vi "Close Log File.vi"(8 "error in (no error)":errorcluster, 11 "PCAP Frame Logger in":refnum<class "PCAP Frame Logger.lvclass">) -> (0 "error out":errorcluster, 3 "PCAP Frame Logger out":refnum<class "PCAP Frame Logger.lvclass">)   [LabVIEW 2020, in "Frame Logging.lvlib" / "PCAP Frame Logger.lvclass"]
uses:
  PCAP Frame Logger.lvclass
  PCAP Frame Logger.lvclass/PCAP Frame Logger.ctl
  <vilib>/Utility/SystemLogging/NI_SystemLogging.lvlib
  libpcaplv/libpcaplv.lvlib
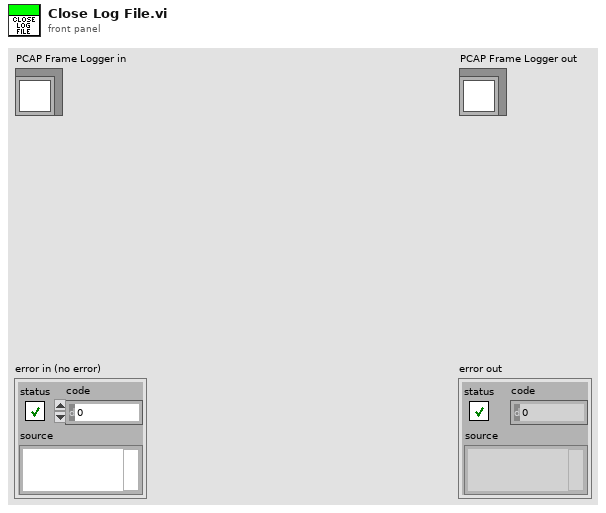
[diagram p1: front panel]
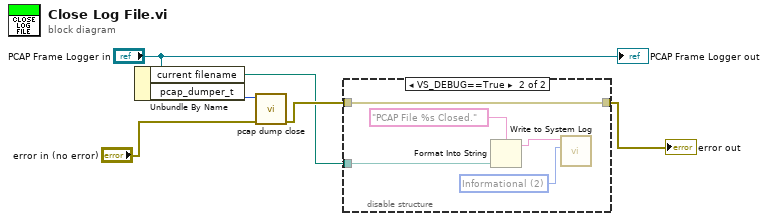
[diagram p0: block diagram]
diagram:
  n1 = Unbundle By Name("PCAP Frame Logger in") -> ("current filename"=w1:path, "pcap_dumper_t"=w3:u64)
  n2 = call "pcap dump close.vi"("error in"="error in (no error)", "pcap_dumper_t in"=w3) -> ("error out"=w2:errorcluster)  [unwired: 9 in]
  n3 = disable-structure shown="VS_DEBUG==True" {
    disable-tunnel: w2 -> [_ w10]
    disable-tunnel: [_ w10] -> w6
    disable-tunnel: w1 -> [_ w7]
    frame condition #0 (active) {
    }
    frame condition #1 {
      w11 = 2 items=["Error", "Warning", "Informational"] ("severity")
      n4 = Format Into String(format string="PCAP File %s Closed.", w7) -> (resulting string=w8:string)  [unwired: 2 in, 1 out]
      n5 = call <vilib>:"Write to System Log.vi"("severity"=w11, "message"=w8) -> ()  [unwired: 9 in, 1 out]
    }
  }
  "error out" <- w6
  "PCAP Frame Logger out" <- "PCAP Frame Logger in"
